vi "CreateUserProject.vi"(4 "Overlay Icon":refnum<class "Icon.lvclass">, 6 "Target Project Name":string, 7 "MetaDataObj":refnum<class "MetaDataObj.lvclass">, 8 "error in (no error)":errorcluster, 9 "Target File Prefix":string, 10 "Target Path":path, 11 "Source Project Path":path) -> (0 "error out":errorcluster, 3 "Project":refnum<vi>)   [LabVIEW 2016, in "NI_NPW_Project Copying.lvlib"]
uses:
  <resource>/dialog/NewProjectWizard/Project Copying/NI_NPW_Project Copying.lvlib
  <vilib>/LabVIEW Icon API/lv_icon/Classes/Icon/Icon.lvclass
  <resource>/dialog/NewProjectWizard/MetaDataObj/MetaDataObj.lvclass
  <resource>/dialog/NewProjectWizard/MetaDataObj/Accessors/CustomVIModes.ctl
  <resource>/dialog/NewProjectWizard/MetaDataObj/MetaDataObj.lvclass/MetaDataObj.ctl
  <resource>/dialog/NewProjectWizard/MetaDataObj/Accessors/Read Panels Open.vi
  <resource>/dialog/NewProjectWizard/MetaDataObj/Accessors/Read Panels Minimized.vi
  <resource>/dialog/NewProjectWizard/MetaDataObj/Accessors/Read Hide Prefix.vi
  <resource>/dialog/NewProjectWizard/MetaDataObj/Accessors/Read Hide Icon Overlay.vi
  <resource>/dialog/NewProjectWizard/MetaDataObj/Accessors/Read Custom VI Mode.vi
  <vilib>/Utility/EditLVProj/Edit LVProj.lvlib
  <resource>/dialog/NewProjectWizard/Icon Overlay/NI_NPW_Icon Overlay.lvlib
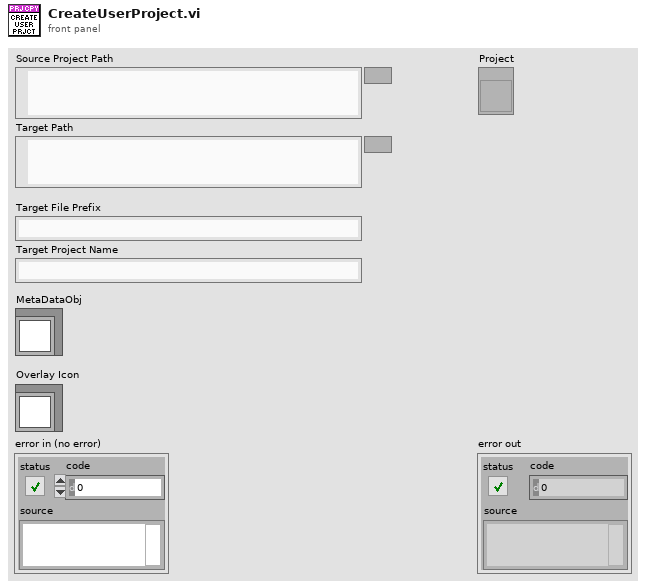
[diagram p1: front panel]
types:
  T1 = typedef "CustomVIModes.ctl" = enum16{"None", "AfterPage1", "AfterPage2WithUI", "AfterPage2NoUI"}
  T2 = typedef "Edit LVProj.lvlib/Library And VI References.ctl" = cluster{"Target Reference":refnum<vi>, "VI References":refnum<vi>[], "Library References":refnum<vi>[]}
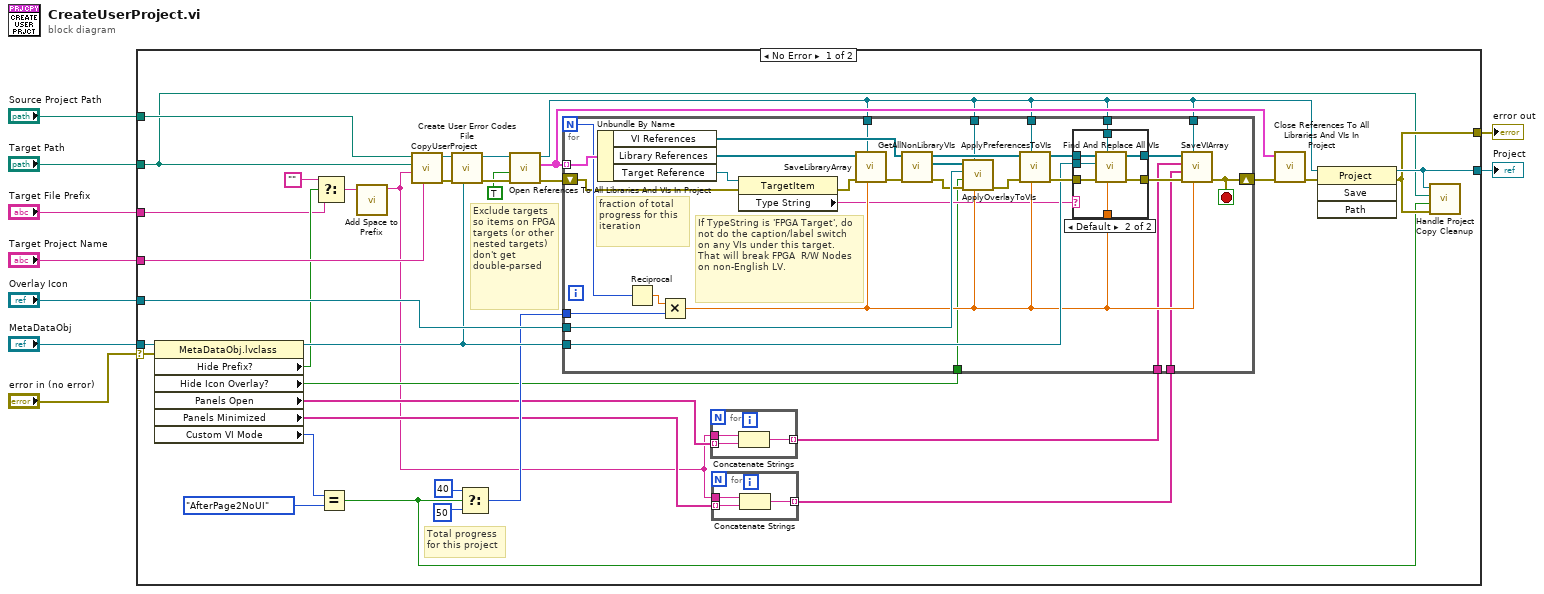
[diagram p0: block diagram]
diagram:
  n1 = case shown="No Error" "error in (no error)" {
    selector: "error in (no error)" -> [w23 w91]
    tunnel: "Overlay Icon" -> [w44 _]
    tunnel: "Source Project Path" -> [w43 _]
    tunnel: "Target Path" -> [w21 _]
    tunnel: "Target Project Name" -> [w42 _]
    tunnel: "MetaDataObj" -> [w40 _]
    tunnel: "Target File Prefix" -> [w12 _]
    tunnel: [w27 _] -> w3
    tunnel: [w22 w91] -> w2
    frame No Error {
      # "Exclude targets so items on FPGA targets (or other nested targets) don't get double-parsed"
      # "Total progress\nfor this project"
      n2 = property class="MetaDataObj.lvclass"(reference=w40, error in=w23) -> (reference out=w38:refnum<class "MetaDataObj.lvclass">, "Hide Prefix?"=w37:bool, "Hide Icon Overlay?"=w19:bool, "Panels Open"=w16:string[], "Panels Minimized"=w14:string[], "Custom VI Mode"=w18:T1)  [unwired: 1 out]
      n3 = Select(t="", s=w37, f=w12) -> (s? t:f=w11:string)
      n4 = Equal?(x=w18, y=CustomVIModes."AfterPage2NoUI") -> (x = y?=w17:bool)
      n5 = call <resource>:"Add Space to Prefix.vi"("Target File Prefix in"=w11) -> ("Target File Prefix out"=w10:string)  [unwired: 10 in]
      n6 = call <resource>:"CopyUserProject.vi"("DNL_Target Project Name"=w42, "DNL_Target File Prefix"=w10, "DNL_Target Path"=w21, "DNL_Source Path"=w43) -> ("error out"=w30:errorcluster, "DNL_New Project Ref"=w35:refnum<vi>)  [unwired: 6 in]
      n7 = call <resource>:"Create User Error Codes File.vi"("MetaDataObj"=w38, "error in (no error)"=w30, "Project"=w35) -> ("error out"=w41:errorcluster, "dup Project"=w39:refnum<vi>)  [unwired: 7 in]
      n8 = Select(t=40, s=w17, f=50) -> (s? t:f=w24:i32)
      n9 = call <vilib>:"Open References To All Libraries And VIs In Project.vi"("error in (no error)"=w41, "Exclude Targets? (F)"=TRUE, "Project in"=w39) -> ("error out"=w34:errorcluster, "VI and Library References"=w31:T2[], "Project out"=w29:refnum<vi>)  [unwired: 6 in]
      n10 = for {
        tunnel: w16 -> [w50] mode=indexing
        tunnel: [w49] -> w15 mode=indexing
        tunnel: w10 -> [w48]
        n11 = Concatenate Strings(w48, w50) -> (w49:string)
      }
      n12 = for {
        tunnel: w14 -> [w47] mode=indexing
        tunnel: [w46] -> w13 mode=indexing
        tunnel: w10 -> [w45]
        n13 = Concatenate Strings(w45, w47) -> (w46:string)
      }
      n14 = for {
        N -> [w62]
        tunnel: w44 -> [w81]
        tunnel: w38 -> [w72]
        tunnel: w31 -> [w79] mode=indexing
        shift-right: [w58] -> w33
        shift-left: w34 -> [w57]
        tunnel: w29 -> [w67]
        tunnel: w29 -> [w66]
        tunnel: w29 -> [w65]
        tunnel: w29 -> [w64]
        tunnel: w29 -> [w63]
        tunnel: w24 -> [w60]
        tunnel: w19 -> [w53]
        tunnel: w15 -> [w52]
        tunnel: w13 -> [w51]
        stop <- w58 stop-if-true
        # "If TypeString is 'FPGA Target', do not do the caption/label switch on any VIs under this target.  That will break FPGA  R/W Nodes on non-English LV."
        # "fraction of total progress for this iteration"
        n15 = Unbundle By Name(w79) -> ("VI References"=w68:refnum<vi>[], "Library References"=w78:refnum<vi>[], "Target Reference"=w54:refnum<vi>)
        n16 = Reciprocal(x=w62) -> (1/x=w61:dbl)
        n17 = Multiply(x=w61, y=w60) -> (x*y=w59:dbl)
        n18 = property class="TargetItem"(reference=w54, error in=w57) -> (error out=w56:errorcluster, "Type String"=w55:string)  [unwired: 1 out]
        n19 = call <resource>:"SaveLibraryArray.vi"("Total Project Progress"=w59, "Project"=w67, "error in (no error)"=w56, "Library References"=w78) -> ("error out"=w70:errorcluster)  [unwired: 7 in]
        n20 = call <resource>:"GetAllNonLibraryVIs.vi"("error in (no error)"=w70, "VI References"=w68) -> ("error out"=w69:errorcluster, "Non-Library VI References"=w76:refnum<vi>[], "dup VI References"=w80:refnum<vi>[])  [unwired: 7 in]
        n21 = call <resource>:"ApplyOverlayToVIs.vi"("Total Iteration Progress"=w59, "Project"=w66, "error in (no error)"=w69, "Hide Overlay?"=w53, "Overlay Icon"=w81, "VIs"=w76) -> ("error out"=w77:errorcluster)  [unwired: 5 in]
        n22 = call <resource>:"ApplyPreferencesToVIs.vi"("Total Iteration Progress"=w59, "Project"=w65, "error in (no error)"=w77, "VIs"=w80) -> ("error out"=w75:errorcluster, "dup VIs"=w73:refnum<vi>[])  [unwired: 6 in]
        n23 = case shown="Default" w55 {
          tunnel: w75 -> [w82 w90]
          tunnel: [w82 w89] -> w74
          tunnel: w73 -> [w83 w88]
          tunnel: w72 -> [_ w87]
          tunnel: [w83 w86] -> w71
          tunnel: w64 -> [_ w85]
          tunnel: w59 -> [_ w84]
          frame "FPGA Target" {
          }
          frame Default {
            n24 = call <resource>:"Find And Replace All VIs.vi"("Total Iteration Progress"=w84, "Project"=w85, "error in (no error)"=w90, "MetaDataObj"=w87, "VI References"=w88) -> ("error out"=w89:errorcluster, "dup VI References"=w86:refnum<vi>[])  [unwired: 5 in]
          }
        }
        n25 = call <resource>:"SaveVIArray.vi"("Total Iteration Progress"=w59, "Project"=w63, "error in (no error)"=w74, "Panels Minimized"=w51, "Panels Open"=w52, "VIs In"=w71) -> ("error out"=w58:errorcluster)  [unwired: 5 in]
      }
      n26 = call <vilib>:"Close References To All Libraries And VIs In Project.vi"("error in (no error)"=w33, "VI and Library References"=w31) -> ("error out"=w32:errorcluster)  [unwired: 9 in]
      n27 = invoke class="Project" method="Save"(reference=w29, error in=w32) -> (reference out=w27:refnum<vi>, error out=w22:errorcluster)  [unwired: 2 in, 2 out]
      n28 = call <resource>:"Handle Project Copy Cleanup.vi"("error in (no error)"=w22, "More Scripting?"=w17, "Target Path"=w21, "Project in"=w27) -> ()  [unwired: 8 in]
    }
    frame Error {
    }
  }
  "Project" <- w3
  "error out" <- w2
